vi "modify channel test.vi"() -> (0 "no err":errorcluster, 3 "mod success":bool)   [LabVIEW 2015, in "DAQmx Module Tests.lvlib"]
doc: "Tests the 'Replace Line' VI."
uses:
  DAQmx Module Tests.lvlib
  <vilib>/NI/Tag Bus Module Framework/channel/TBM channel.lvclass/TBM channel.ctl
  <vilib>/NI/Tag Bus Module Framework/channel/channel classification.ctl
  <vilib>/NI/Tag Bus/tag/tag descriptor.lvclass/tag descriptor.ctl
  <vilib>/NI/Tag Bus Module Framework/channel/Read channel classification.vi
  <vilib>/NI/Tag Bus Module Framework/channel/Write channel classification.vi
  module/configuration/Daqmx Module configuration.lvclass
  <vilib>/NI/Tag Bus Module Framework/channel/TBM channel.lvclass
  <vilib>/NI/Tag Bus/tag/tag descriptor.lvclass
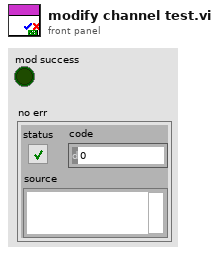
[diagram p1: front panel]
types:
  T1 = typedef "DAQmx Module Configuration.lvclass/Line.ctl" = cluster{"Channel Array":refnum<class "TBM channel.lvclass">[], "Physical Channel":string, "Measurement Type":T2, "Parameters":T3}
  T2 = typedef "DAQmx Module Configuration.lvclass/Measurement Type.ctl" = enum16{"Digital Input", "Digital Output", "Voltage Input", "Voltage Output", "Current Input", "Current Output", "RTD", "Thermocouple", "Strain", "PWM"}
  T3 = typedef "DAQmx Module Configuration.lvclass/Parameters.ctl" = cluster{"Digital Config":cluster{"Invert Lines?":bool}, "Voltage Config":cluster{"Maximum Value (V)":dbl, "Minimum Value (V)":dbl, "in terminal configuration (V)":i32, "out terminal configuration (V)":i32}, "Current Config":cluster{"Maximum Value (A)":dbl, "Minimum Value (A)":dbl, "shunt resistor location":i32, "input terminal configuration (C)":i32, "external shunt resistor value":dbl}, "RTD Config":cluster{"Maximum Value (°C)":dbl, "Minimum Value (°C)":dbl, "resistance configuration":i32, "r0":dbl, "current excitation value":dbl, "rtd type":i32, "current excitation source":i32}, "Thermocouple Config":cluster{"Minimum Value (C)":dbl, "Maximum Value (C)":dbl, "thermocouple type":i32, "cjc source":i32, "cjc value":dbl}, "Strain Config":cluster{"Maximum Value":dbl, "Minimum Value":dbl, "bridge information":cluster{"strain configuration":i32, "lead wire resistance":dbl, "initial bridge voltage":dbl, "voltage excitation source":i32, "voltage excitation value":dbl}, "strain gage information":cluster{"gage factor":dbl, "nominal gage resistance":dbl, "poisson ratio":dbl}}, "PWM Config":cluster{"Idle State":bool}}
  T4 = typedef "TBM channel.lvclass/channel classification.ctl" = enum16{"input data", "output data", "processing parameter", "processing result"}
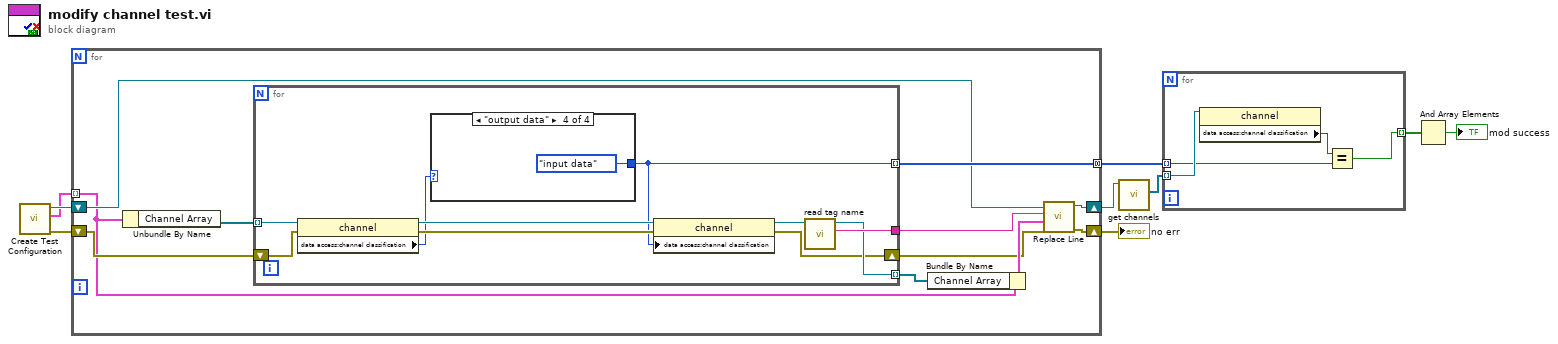
[diagram p0: block diagram]
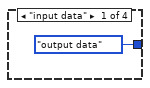
[diagram p2: hidden frame]
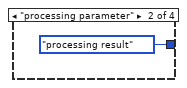
[diagram p3: hidden frame]
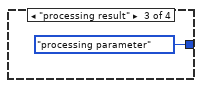
[diagram p4: hidden frame]
diagram:
  n1 = call "Create Test Configuration.vi"() -> ("error out"=w1:errorcluster, "Line Array"=w2:T1[], "Module Configuration"=w3:refnum<class "Daqmx Module configuration.lvclass">)  [unwired: 6 in, 3 out]
  n2 = for {
    shift-right: [w16] -> w9
    shift-left: w3 -> [w15]
    shift-right: [w17] -> w8
    shift-left: w1 -> [w20]
    tunnel: w2 -> [w14] mode=indexing
    tunnel: [w19] -> w4 mode=concatenating
    n3 = Unbundle By Name(w14) -> ("Channel Array"=w18:refnum<class "TBM channel.lvclass">[])
    n4 = for {
      tunnel: [w26] -> w19 mode=indexing
      tunnel: w18 -> [w25] mode=indexing
      tunnel: [w24] -> w12
      tunnel: [w22] -> w11 mode=indexing
      shift-right: [w21] -> w10
      shift-left: w20 -> [w30]
      n5 = property class="channel"(reference=w25, error in=w30) -> (reference out=w28:refnum<class "TBM channel.lvclass">, error out=w29:errorcluster, "data access:channel classification"=w27:T4)
      n6 = case shown="\"output data\"" w27 {
        tunnel: [channel_classification."output data" ("channel classification") channel_classification."processing result" ("channel classification") channel_classification."processing parameter" ("channel classification") channel_classification."input data" ("channel classification")] -> w26
        frame "input data" {
        }
        frame "processing parameter" {
        }
        frame "processing result" {
        }
        frame "output data" {
        }
      }
      n7 = property class="channel"(reference=w28, error in=w29, "data access:channel classification"=w26) -> (reference out=w23:refnum<class "TBM channel.lvclass">, error out=w21:errorcluster)
      n8 = call <vilib>:"read tag name.vi"("system tag in"=w23) -> ("name"=w24:string, "system tag out"=w22:refnum<class "TBM channel.lvclass">)  [unwired: 8 in, 1 out]
    }
    n9 = Bundle By Name(cluster=w14, "Channel Array"=w11) -> (w13:T1)
    n10 = call "Replace Line.vi"("error in"=w10, "New Line"=w13, "Line Name"=w12, "Daqmx Module configuration in"=w15) -> ("error out"=w17:errorcluster, "Daqmx Module configuration out"=w16:refnum<class "Daqmx Module configuration.lvclass">)  [unwired: 5 in, 1 out]
  }
  "no err" <- w8
  n11 = call-dynamic "get channels.vi"("Daqmx Module configuration in"=w9) -> ("channels"=w7:refnum<class "TBM channel.lvclass">[])  [unwired: 9 in, 1 out]
  n12 = for {
    tunnel: w7 -> [w38] mode=indexing
    tunnel: [w35] -> w6 mode=indexing
    tunnel: w4 -> [w37] mode=indexing
    n13 = property class="channel"(reference=w38) -> ("data access:channel classification"=w36:T4)  [unwired: 1 in, 2 out]
    n14 = Equal?(x=w36, y=w37) -> (x = y?=w35:bool)
  }
  n15 = And Array Elements(Boolean array=w6) -> (logical AND=→"mod success":bool)
